vi "GetSerializationDetails.vi"(8 "error in (no error)":errorcluster, 11 "ClassConverter in":refnum<class "ClassConverter.lvclass">) -> (0 "error out":errorcluster, 1 "ID":string, 2 "FileType":T1, 3 "ClassConverter out":refnum<class "ClassConverter.lvclass">, 4 "ComponentsSerialized":string)   [LabVIEW 2017, in "ClassConverter.lvclass"]
uses:
  ClassConverter.lvclass
  SupportedFileTypes.ctl
  Helpers/DirectoryMetadata/DirectoryMetadata.lvclass
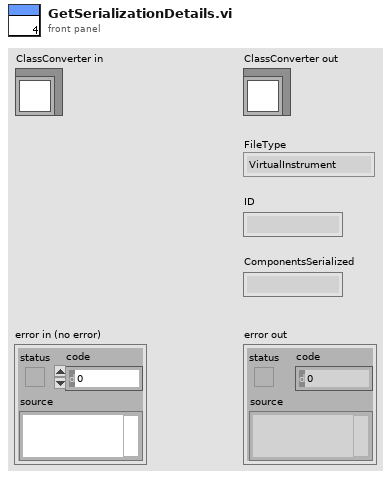
[diagram p1: front panel]
types:
  T1 = typedef "SupportedFileTypes.ctl" = enum16{"VirtualInstrument", "Class", "Project"}
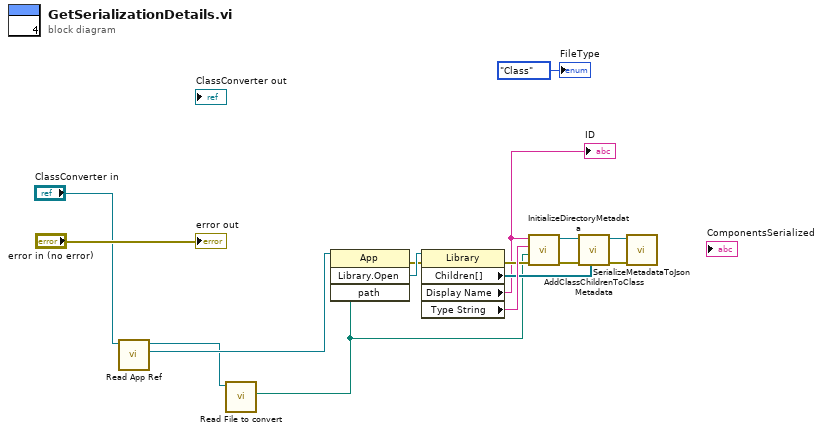
[diagram p0: block diagram]
diagram:
  n1 = call-dynamic "Read App Ref.vi"("FileConverterBase in"="ClassConverter in") -> ("App Ref"=w4:refnum<vi>, "FileConverterBase out"=w3:refnum<class "ClassConverter.lvclass">)  [unwired: 8 in, 1 out]
  n2 = call-dynamic "Read File to convert.vi"("FileConverterBase in"=w3) -> ("Input File Path"=w2:path)  [unwired: 8 in, 2 out]
  n3 = invoke class="App" method="Library.Open"(reference=w4, "path"=w2) -> (error out=w13:errorcluster, "Open Library"=w14:refnum<vi>)  [unwired: 2 in, 2 out]
  n4 = property class="Library"(reference=w14, error in=w13) -> (error out=w8:errorcluster, "Children[]"=w11:refnum<vi>[], "Display Name"=w1:string, "Type String"=w12:string)  [unwired: 1 out]
  "ID" <- w1
  n5 = call "InitializeDirectoryMetadata.vi"("Error in"=w8, "Path"=w2, "Type"=w12, "ID"=w1) -> ("Error out"=w7:errorcluster, "DirectoryMetadata instance"=w10:refnum<data-value>)  [unwired: 6 in]
  n6 = call "AddClassChildrenToClassMetadata.vi"("Children[]"=w11, "error in"=w7, "ClassMetadata instance"=w10) -> ("error out"=w6:errorcluster, "ClassMetadata instance out"=w9:refnum<data-value>)  [unwired: 7 in]
  n7 = call "SerializeMetadataToJson.vi"("error in (no error)"=w6, "head in"=w9) -> ()  [unwired: 7 in, 3 out]
  "error out" <- "error in (no error)"
  "FileType" <- SupportedFileTypes."Class" ("FileType")
